vi "Configure FM Internal [FM] Core.vi"(7 "modulation waveform (Sine)":i32(ring)=1 items=["Sine"=1, "Square"=2, "Triangle"=3, "Ramp Up"=4, "Ramp Down"=5], 8 "error in (no error)":errorcluster, 9 "modulation frequency (1000 Hz)":dbl[unit]=1000.0 format="%^.2e", 10 "peak deviation (100 Hz)":dbl[unit]=100.0 format="%^.2e", 11 "IVI_Fgen in":refnum<class "IVI_Fgen.lvclass">) -> (0 "error out":errorcluster, 3 "IVI_Fgen out":refnum<class "IVI_Fgen.lvclass">)   [LabVIEW 2013, in "IVI_Fgen.lvlib" / "IVI_Fgen.lvclass"]
doc: "This VI configures the properties that control the function generator's internal frequency modulation source. These properties are the peak deviation, waveform, and frequency.\n\nNotes:\n\n(1) This VI is part of the IviFgenModulateFM [FM] extension group."
uses:
  IVI_Fgen.lvclass
  IVI_Fgen.lvclass/IVI_Fgen.ctl
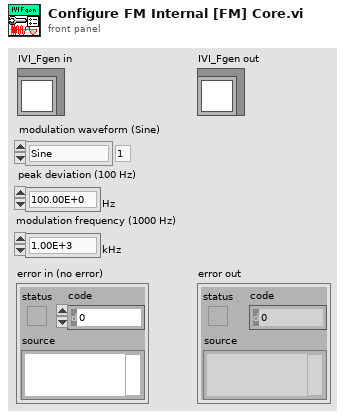
[diagram p1: front panel]
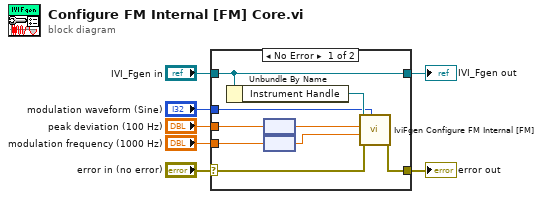
[diagram p0: block diagram]
diagram:
  n1 = case shown="No Error" "error in (no error)" {
    selector: "error in (no error)" -> [w14 w18]
    tunnel: [w13 w18] -> w6
    tunnel: [w16 w17] -> w4
    tunnel: "IVI_Fgen in" -> [w16 w17]
    tunnel: "modulation waveform (Sine)" -> [w12 _]
    tunnel: "peak deviation (100 Hz)" -> [w11 _]
    tunnel: "modulation frequency (1000 Hz)" -> [w9 _]
    frame No Error {
      n2 = Unbundle By Name(w16) -> ("Instrument Handle"=w15:refnum<k15>)
      n3 = node(w11) -> (w10:dbl)
      n4 = node(w9) -> (w8:dbl)
      n5 = call <vilib>:"IviFgen Configure FM Internal [FM].vi"("modulation waveform (Sine)"=w12, "error in (no error)"=w14, "modulation frequency (1000 Hz)"=w8, "peak deviation (100 Hz)"=w10, "instrument handle"=w15) -> ("error out"=w13:errorcluster)  [unwired: 5 in, 1 out]
    }
    frame Error {
    }
  }
  "error out" <- w6
  "IVI_Fgen out" <- w4
